vi "Array Size and Index.vi"() -> ()   [LabVIEW 2024]
panel:
  out "size(s)":i32
  in  "Array to find index":dbl
  out "Res":dbl
  out "Array 2":dbl[](array[slide]) scale=0.0..20.0
  in  "Array":dbl[](array[numeric])
  # "Overview:\nIn this VI a few array elements are used to find the array size and te Index array inorder to find the value of the element find \nin that particular position.\nInstructions:\n1. Give the values in the array and the position you want to find the index.\n2. Run the VI."
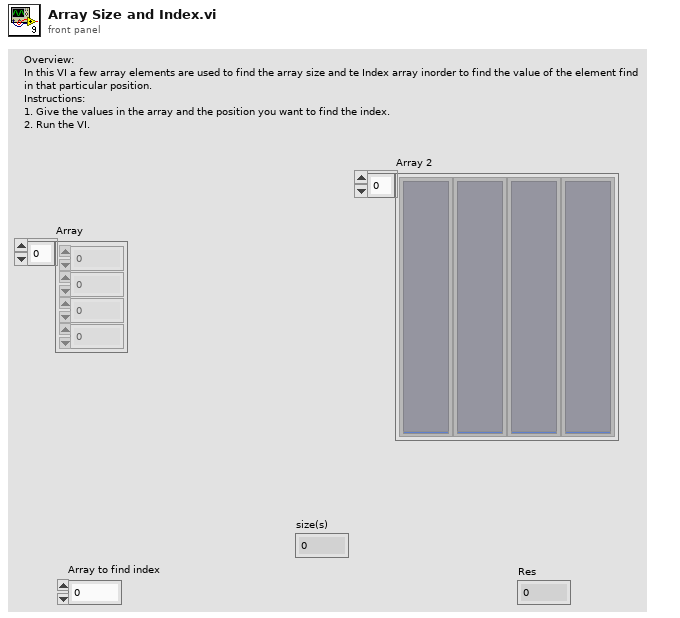
[diagram p1: front panel]
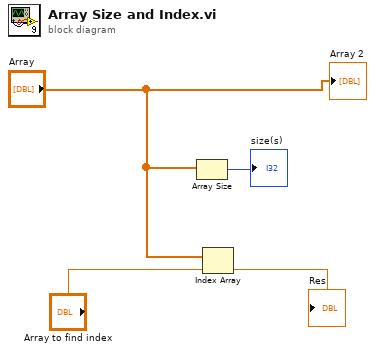
[diagram p0: block diagram]
diagram:
  n1 = Array Size(array="Array") -> (size(s)=→"size(s)":i32)
  n2 = Index Array "Index Array"(array="Array", index="Array to find index") -> (element=→"Res":dbl)
  "Array 2" <- "Array"
